vi "jVision.vi"() -> ()   [LabVIEW 2013]
uses:
  <vilib>/userDefined/High Color/IMAQdx.ctl
  Controls/States.ctl
  <vilib>/vision/driver/NI_Vision_Acquisition_Software.lvlib
  <resource>/objmgr/imaqdx.rc
panel:
  in  "Auto Clear":bool=TRUE
  out "User Notes File Name":path
  in  "Experiment Notes":string
  in  "Set Camera Properties":bool=TRUE
  in  "SyncOutSource":string(combo)="FreeRun"
  in  "SyncOutSelector":string(combo)="FrameStart"
  out "Max. Frame Rate":u32
  out "Cam Session":T1 caption="Session Out"
  in  "File Name Prefix":string="Rawdata "
  in  "File Path":path=path "E:/Rawdata"
  in  "Width":u32=1920 min=1 max=1920
  in  "Height":u32=1080 min=1 max=1080
  out "Stopped":bool
  in  "Exp. Time (S)":u32=60
  out "Frames to Acquire":u32
  in  "Set Frame Rate":u32=25 max=60
  in  "Start":bool
  out "Exp Time":dbl caption="Elapsed Time (s)"
  out "Frame Rate":dbl format="%#_4f"
  in  "Camera ID":T1="cam1"
  out "Frames Acquired":i32
  out "JVision - Release F":T2(plugin-control)
  in  "Stop Button":bool
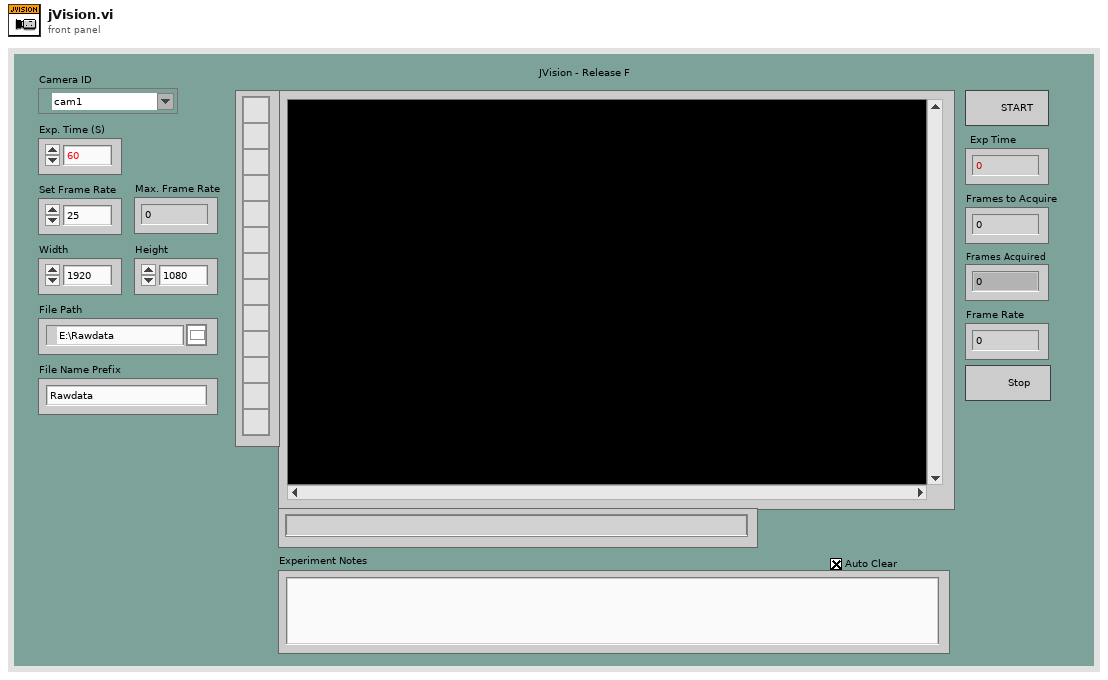
[diagram p1: front panel]
types:
  T1 = typedef "IMAQdx.ctl" = refnum<k21>
  T2 = typedef "IMAQ Image.ctl" = refnum<image>
  T3 = typedef "States.ctl" = enum16{"Initialize", "Wait for Start", "Set Param", "Initialize Acquisition", "Run Acquisition", "Stop"}
  T4 = enum16{"open", "replace", "create", "open or create", "replace or create", "replace or create with confirmation"}
  T5 = typedef "Image Type" = u32
  T6 = enum8{"Enabled", "Disabled", "Disabled and Grayed Out"}
  T7 = typedef "AviRefnum.ctl" = refnum<k1>
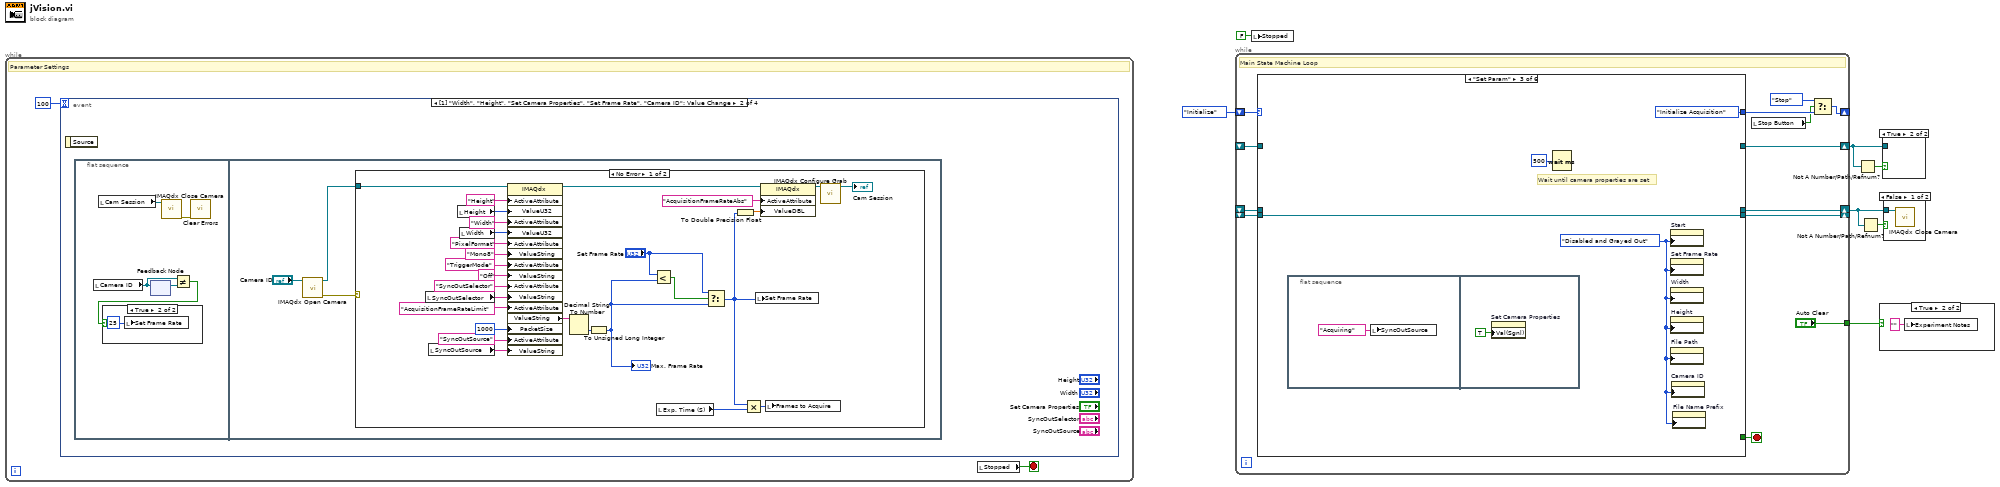
[diagram p0: block diagram]
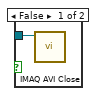
[diagram p4: hidden frame]
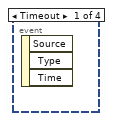
[diagram p5: hidden frame]
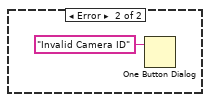
[diagram p7: hidden frame]
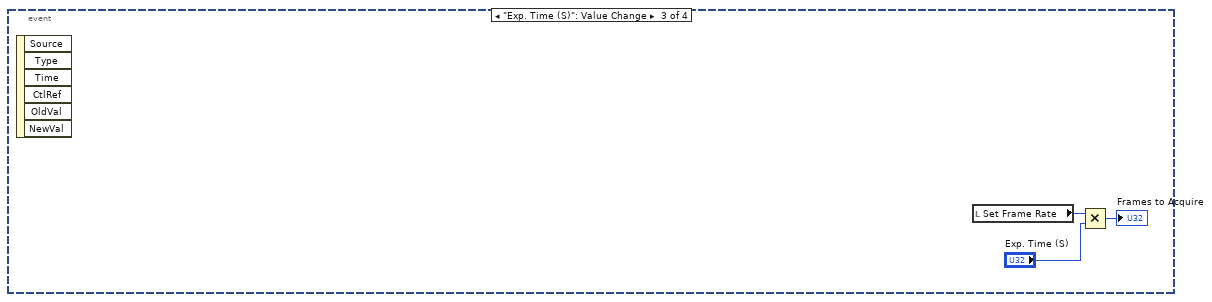
[diagram p8: hidden frame]
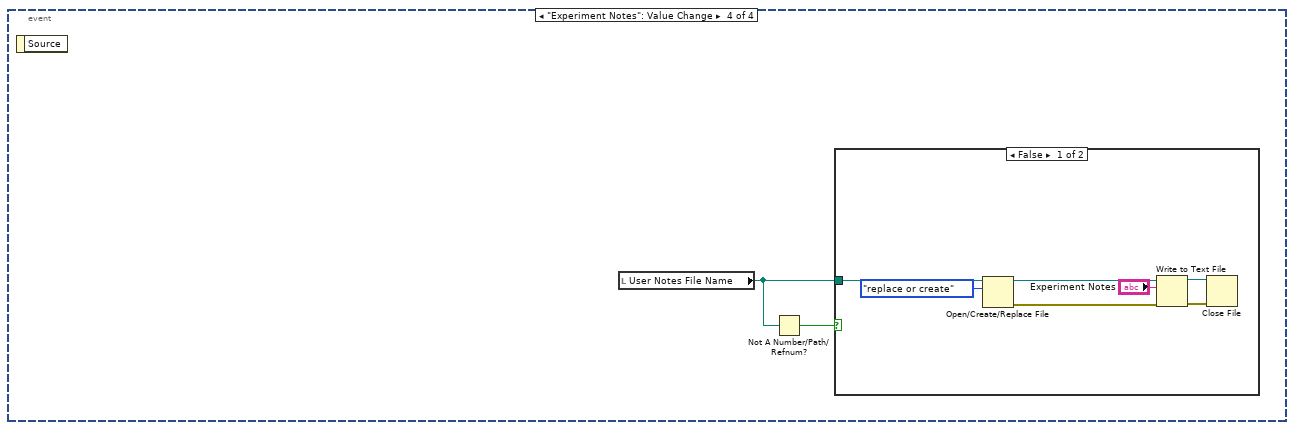
[diagram p9: hidden frame]
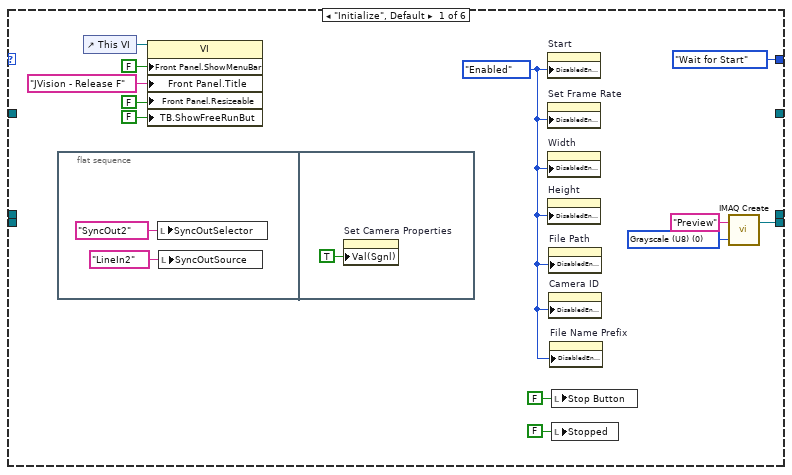
[diagram p11: hidden frame]
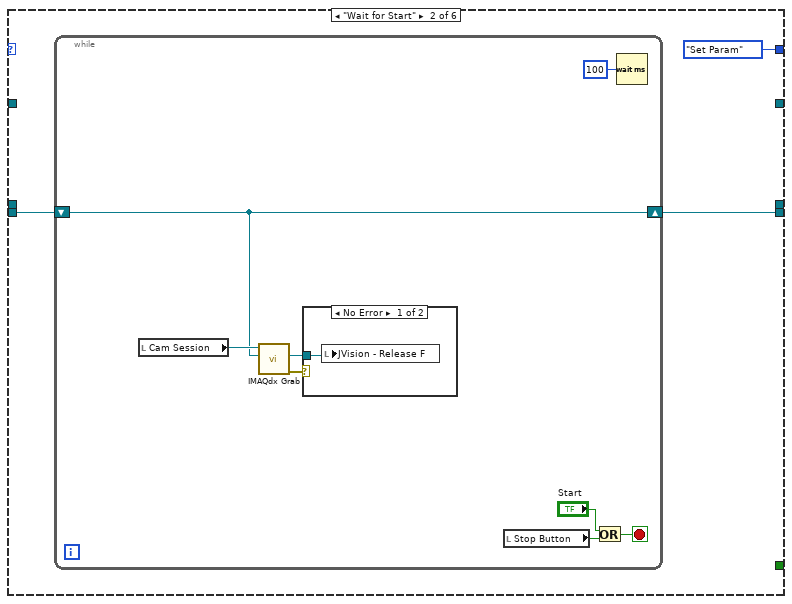
[diagram p12: hidden frame]
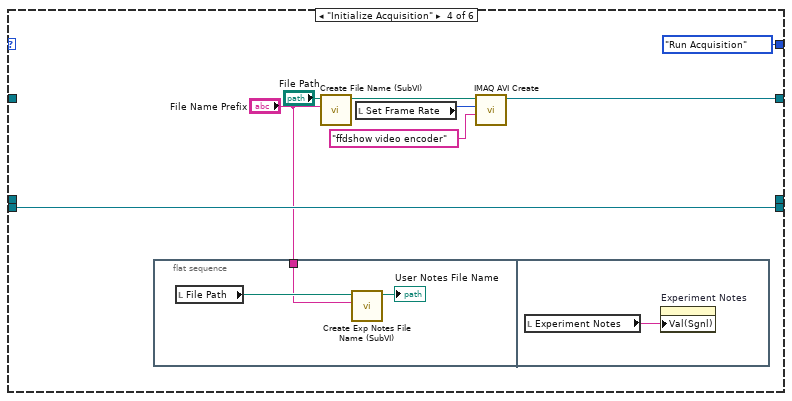
[diagram p14: hidden frame]
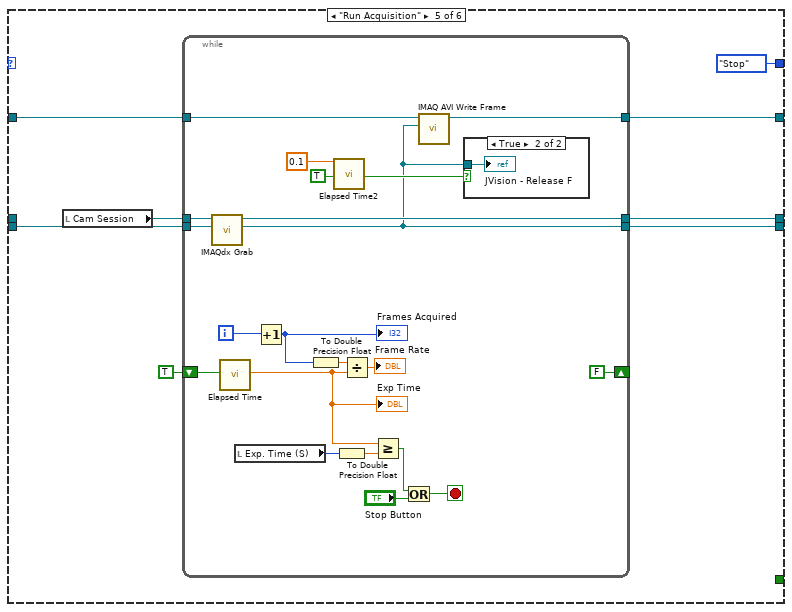
[diagram p15: hidden frame]
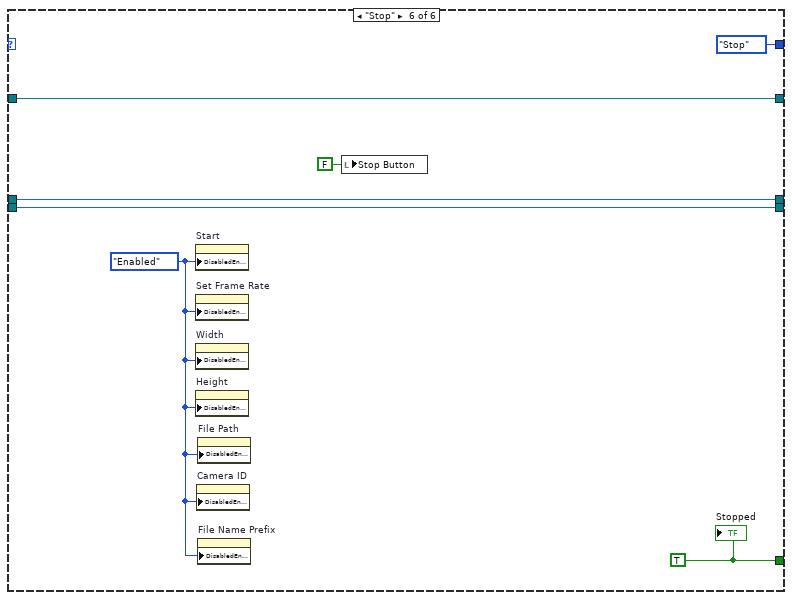
[diagram p17: hidden frame]
diagram:
  n1 = while {
    stop <- w9 stop-if-true
    # "Parameter Settings"
    n2 = event shown="[1] \"Width\", \"Height\", \"Set Camera Properties\", \"Set Frame Rate\", \"Camera ID\": Value Change" {
      selector: _ -> [_ _ _ _]
      dyn-events: _ -> [_ _ _ _]
      timeout: 100 -> [_ _ _ _]
      event Timeout {
        n3 = event-data() -> ()  [unwired: 1 in, 3 out]
      }
      event "Width", "Height", "Set Camera Properties", "Set Frame Rate": Value Change {
        n4 = event-data() -> ()  [unwired: 1 in, 1 out]
        n5 = flat-sequence {
          frame #0 {
            n6 = local read "Camera ID"() -> (w11:T1)
            n7 = local read "Cam Session"() -> (w13:T1)
            n8 = feedback #1() -> (w12:T1)  [unwired: 1 in]
            n9 = feedback-in #1(w11) -> ()
            n10 = call <vilib>:"IMAQdx Close Camera.vi"("Session In"=w13) -> ("error out"=w14:errorcluster)  [unwired: 10 in]
            n11 = Not Equal?(x=w11, y=w12) -> (x != y?=w10:bool)
            n12 = case shown="True" w10 {
              frame False {
              }
              frame True {
                n13 = local write "Set Frame Rate"(u32 25 ("Set Frame Rate")) -> ()
              }
            }
            n14 = call <vilib>:"Clear Errors.vi"("error in (no error)"=w14) -> ()  [unwired: 6 in, 1 out]
          }
          frame #1 {
            n15 = call <vilib>:"IMAQdx Open Camera.vi"("Session In"="Camera ID") -> ("error out"=w17:errorcluster, "Session Out"=w16:T1)  [unwired: 9 in]
            n16 = case shown="No Error" w17 {
              tunnel: w16 -> [w19 _]
              frame No Error {
                n17 = local read "SyncOutSelector"() -> (w25:string)
                n18 = local read "SyncOutSource"() -> (w24:string)
                n19 = local read "Height"() -> (w44:u32)
                n20 = local read "Width"() -> (w43:u32)
                n21 = property class="IMAQdx"(reference=w19, "ActiveAttribute"="Height", "ValueU32"=w44, "ActiveAttribute"="Width", "ValueU32"=w43, "ActiveAttribute"="PixelFormat", "ValueString"="Mono8" ("ActiveAttribute"), "ActiveAttribute"="TriggerMode", "ValueString"="Off", "ActiveAttribute"="SyncOutSelector", "ValueString"=w25, "ActiveAttribute"="AcquisitionFrameRateLimit", "PacketSize"=u32 1000, "ActiveAttribute"="SyncOutSource", "ValueString"=w24) -> (reference out=w32:T1, "ValueString"=w36:string)  [unwired: 1 in, 1 out]
                n22 = Decimal String To Number(string=w36) -> (number=w37:i32)  [unwired: 2 in, 1 out]
                n23 = To Unsigned Long Integer(number=w37) -> (unsigned 32bit integer=w28:u32)
                "Max. Frame Rate" <- w28
                n24 = Less?(x="Set Frame Rate", y=w28) -> (x < y?=w34:bool)
                n25 = local read "Exp. Time (S)"() -> (w22:u32)
                n26 = Select(t="Set Frame Rate", s=w34, f=w28) -> (s? t:f=w21:u32)
                n27 = To Double Precision Float(number=w21) -> (double precision float=w29:dbl)
                n28 = Multiply(x=w21, y=w22) -> (x*y=w23:u32)
                n29 = local write "Set Frame Rate"(w21) -> ()
                n30 = property class="IMAQdx"(reference=w32, "ActiveAttribute"="AcquisitionFrameRateAbs", "ValueDBL"=w29) -> (reference out=w31:T1)  [unwired: 1 in, 1 out]
                n31 = local write "Frames to Acquire"(w23) -> ()
                n32 = call <vilib>:"IMAQdx Configure Grab.vi"("Session In"=w31) -> ("Session Out"=→"Cam Session":T1)  [unwired: 9 in, 1 out]
              }
              frame Error {
                n33 = One Button Dialog(message="Invalid Camera ID") -> ()  [unwired: 1 in, 1 out]
              }
            }
          }
        }
      }
      event "Exp. Time (S)": Value Change {
        n34 = event-data() -> ()  [unwired: 1 in, 6 out]
        n35 = local read "Set Frame Rate"() -> (w50:u32)
        n36 = Multiply(x=w50, y="Exp. Time (S)") -> (x*y=→"Frames to Acquire":u32)
      }
      event "Experiment Notes": Value Change {
        n37 = event-data() -> ()  [unwired: 1 in, 1 out]
        n38 = local read "User Notes File Name"() -> (w52:path)
        n39 = Not A Number/Path/Refnum?(number/path/refnum=w52) -> (NaN/Path/Refnum?=w51:bool)
        n40 = case shown="False" w51 {
          tunnel: w52 -> [w53 _]
          frame False {
            n41 = Open/Create/Replace File(file path (use dialog)=w53, operation (0:open)=T4."replace or create") -> (refnum out=w57:refnum<file>, error out=w58:errorcluster)  [unwired: 4 in, 1 out]
            n42 = Write to Text File(file (use dialog)=w57, text="Experiment Notes", error in=w58) -> (refnum out=w54:refnum<file>, error out=w55:errorcluster)  [unwired: 1 in, 1 out]
            n43 = Close File(refnum=w54, error in=w55) -> ()  [unwired: 2 out]
          }
          frame True {
          }
        }
      }
    }
    n44 = local read "Stopped"() -> (w9:bool)
  }
  n45 = while {
    shift-right: [w63] -> _
    shift-left: States."Initialize" ("Enum") -> [w71]
    shift-right: [w70] -> _
    shift-left: _ -> [w69]
    shift-right: [w68] -> w4
    shift-left: _ -> [w67]
    shift-right: [w66] -> w6
    shift-left: _ -> [w65]
    tunnel: ["Auto Clear"] -> w1
    stop <- w64 stop-if-true
    # "Main State Machine Loop"
    n46 = case shown="\"Set Param\"" w71 {
      tunnel: [States."Wait for Start" ("Enum") States."Set Param" ("Enum") States."Initialize Acquisition" ("Enum") States."Run Acquisition" ("Enum") States."Stop" ("Enum") States."Stop" ("Enum")] -> w72
      tunnel: [w81 w88 w102 w107 w119 w152] -> w70
      tunnel: w69 -> [_ w89 w102 w107 w123 w152]
      tunnel: [_ _ _ _ w120 w151] -> w68
      tunnel: w67 -> [_ _ _ _ _ w151]
      tunnel: [_ _ _ w108 w121 w153] -> w66
      tunnel: w65 -> [_ _ _ _ w124 w153]
      tunnel: [_ _ _ _ _ w149] -> w64
      frame "Initialize", Default {
        w83 = T5 0 items=["Grayscale (U8)", "Grayscale (I16)", "Grayscale (SGL)", "Complex (CSG)", "RGB (U32)", "HSL (U32)", "RGB (U64)", "Grayscale (U16)"] ("Image Type")
        w80 = T6."Enabled" ("Disabled")
        n47 = flat-sequence {
          frame #0 {
            n48 = local write "SyncOutSelector"("SyncOut2" ("SyncOutSelector")) -> ()
            n49 = local write "SyncOutSource"("LineIn2" ("SyncOutSource")) -> ()
          }
          frame #1 {
            n50 = property on="Set Camera Properties" class="Bool (strict)"("Val(Sgnl)"=TRUE ("Value (Signaling)")) -> ()  [unwired: 2 in, 2 out]
          }
        }
        n51 = control-ref of="This VI"() -> (w79:refnum<vi>)
        n52 = property class="VI"(reference=w79, "Front Panel.ShowMenuBar"=FALSE ("Front Panel Window:Show Menu Bar"), "Front Panel.Title"="JVision - Release F" ("Front Panel Window:Title"), "Front Panel.Resizeable"=FALSE ("Front Panel Window:Resizable"), "TB.ShowFreeRunBut"=FALSE ("Tool Bar:Show Free Run Button")) -> ()  [unwired: 1 in, 2 out]
        n53 = property on="Start" class="Bool"("DisabledEnum"=w80) -> ()  [unwired: 2 in, 2 out]
        n54 = property on="Set Frame Rate" class="DigNum (strict)"("DisabledEnum"=w80) -> ()  [unwired: 2 in, 2 out]
        n55 = property on="Width" class="DigNum (strict)"("DisabledEnum"=w80) -> ()  [unwired: 2 in, 2 out]
        n56 = property on="Height" class="DigNum (strict)"("DisabledEnum"=w80) -> ()  [unwired: 2 in, 2 out]
        n57 = property on="File Path" class="Path"("DisabledEnum"=w80) -> ()  [unwired: 2 in, 2 out]
        n58 = property on="Camera ID" class="IMAQdx (strict)"("DisabledEnum"=w80) -> ()  [unwired: 2 in, 2 out]
        n59 = property on="File Name Prefix" class="Str"("DisabledEnum"=w80) -> ()  [unwired: 2 in, 2 out]
        n60 = local write "Stop Button"(FALSE ("Stop Button")) -> ()
        n61 = local write "Stopped"(FALSE ("Stopped")) -> ()
        n62 = call "IMAQ Create"("Image Name"="Preview", "Image Type"=w83) -> ("New Image"=w81:T2)  [unwired: 3 in, 1 out]
      }
      frame "Wait for Start" {
        n63 = while {
          shift-right: [w91] -> w88
          shift-left: w89 -> [w91]
          stop <- w95 stop-if-true
          n64 = local read "Cam Session"() -> (w94:T1)
          n65 = call <vilib>:"IMAQdx Grab.vi"("Image In"=w91, "Session In"=w94) -> ("error out"=w93:errorcluster, "Image Out"=w92:T2)  [unwired: 6 in, 2 out]
          n66 = case shown="No Error" w93 {
            tunnel: w92 -> [w99 _]
            frame No Error {
              n67 = local write "JVision - Release F"(w99) -> ()
            }
            frame Error {
            }
          }
          n68 = local read "Stop Button"() -> (w96:bool)
          n69 = Or(x="Start", y=w96) -> (x .or. y?=w95:bool)
          n70 = Wait (ms)(milliseconds to wait=u32 100) -> ()  [unwired: 1 out]
        }
      }
      frame "Set Param" {
        w101 = T6."Disabled and Grayed Out" ("Disabled")
        # "Wait until camera properties are set"
        n71 = flat-sequence {
          frame #0 {
            n72 = local write "SyncOutSource"("Acquiring" ("SyncOutSource")) -> ()
          }
          frame #1 {
            n73 = property on="Set Camera Properties" class="Bool (strict)"("Val(Sgnl)"=TRUE ("Value (Signaling)")) -> ()  [unwired: 2 in, 2 out]
          }
        }
        n74 = Wait (ms)(milliseconds to wait=u32 500) -> ()  [unwired: 1 out]
        n75 = property on="Start" class="Bool"("DisabledEnum"=w101) -> ()  [unwired: 2 in, 2 out]
        n76 = property on="Set Frame Rate" class="DigNum (strict)"("DisabledEnum"=w101) -> ()  [unwired: 2 in, 2 out]
        n77 = property on="Width" class="DigNum (strict)"("DisabledEnum"=w101) -> ()  [unwired: 2 in, 2 out]
        n78 = property on="Height" class="DigNum (strict)"("DisabledEnum"=w101) -> ()  [unwired: 2 in, 2 out]
        n79 = property on="File Path" class="Path"("DisabledEnum"=w101) -> ()  [unwired: 2 in, 2 out]
        n80 = property on="Camera ID" class="IMAQdx (strict)"("DisabledEnum"=w101) -> ()  [unwired: 2 in, 2 out]
        n81 = property on="File Name Prefix" class="Str"("DisabledEnum"=w101) -> ()  [unwired: 2 in, 2 out]
      }
      frame "Initialize Acquisition" {
        n82 = flat-sequence {
          tunnel: "File Name Prefix" -> [w114]
          frame #0 {
            n83 = local read "File Path"() -> (w116:path)
            n84 = call "Create Exp Notes File Name (SubVI).vi"("File Name Prefix"=w114, "File Path"=w116) -> ("File Name"=→"User Notes File Name":path)  [unwired: 9 in]
          }
          frame #1 {
            n85 = local read "Experiment Notes"() -> (w117:string)
            n86 = property on="Experiment Notes" class="Str"("Val(Sgnl)"=w117) -> ()  [unwired: 2 in, 2 out]
          }
        }
        n87 = call "Create File Name (SubVI).vi"("File Name Prefix"="File Name Prefix", "File Path"="File Path") -> ("File Name"=w111:path)  [unwired: 9 in]
        n88 = local read "Set Frame Rate"() -> (w113:u32)
        n89 = call "IMAQ AVI Create"("Compression Filter"="ffdshow video encoder", "Frames Per Second"=w113, "AVI Path"=w111) -> ("Avi Refnum"=w108:T7)  [unwired: 7 in, 1 out]
      }
      frame "Run Acquisition" {
        n90 = local read "Cam Session"() -> (w118:T1)
        n91 = while {
          tunnel: w118 -> [w145]
          tunnel: w123 -> [w144]
          tunnel: [w143] -> w120
          shift-right: [FALSE] -> _
          shift-left: TRUE -> [w140]
          tunnel: w124 -> [w129]
          tunnel: [w130] -> w121
          tunnel: [w128] -> w119
          i -> [w126]
          stop <- w142 stop-if-true
          n92 = call <vilib>:"IMAQdx Grab.vi"("Image In"=w144, "Session In"=w145) -> ("Image Out"=w128:T2, "Session Out"=w143:T1)  [unwired: 6 in, 2 out]
          n93 = call "Elapsed Time"("Reset"=w140) -> ("Elapsed Time (s)"=w131:dbl)  [unwired: 11 in, 7 out]
          "Exp Time" <- w131
          n94 = local read "Exp. Time (S)"() -> (w136:u32)
          n95 = Increment(x=w126) -> (x+1=w127:i32)
          "Frames Acquired" <- w127
          n96 = To Double Precision Float(number=w127) -> (double precision float=w137:dbl)
          n97 = call "Elapsed Time2"("Time Target (s)"=0.1, "Auto Reset"=TRUE) -> ("Time has Elapsed"=w133:bool)  [unwired: 10 in, 7 out]
          n98 = To Double Precision Float(number=w136) -> (double precision float=w135:dbl)
          n99 = Divide(x=w137, y=w131) -> (x/y=→"Frame Rate":dbl)
          n100 = Greater Or Equal?(x=w131, y=w135) -> (x >= y?=w141:bool)
          n101 = Or(x=w141, y="Stop Button") -> (x .or. y?=w142:bool)
          n102 = call "IMAQ AVI Write Frame"("Image"=w128, "Avi Refnum"=w129) -> ("Avi Refnum (duplicate)"=w130:T7)  [unwired: 8 in, 1 out]
          n103 = case shown="True" w133 {
            tunnel: w128 -> [_ w147]
            frame False {
            }
            frame True {
              "JVision - Release F" <- w147
            }
          }
        }
      }
      frame "Stop" {
        w148 = T6."Enabled" ("Disabled")
        w149 = TRUE
        n104 = property on="Start" class="Bool"("DisabledEnum"=w148) -> ()  [unwired: 2 in, 2 out]
        n105 = property on="Set Frame Rate" class="DigNum (strict)"("DisabledEnum"=w148) -> ()  [unwired: 2 in, 2 out]
        n106 = property on="Width" class="DigNum (strict)"("DisabledEnum"=w148) -> ()  [unwired: 2 in, 2 out]
        n107 = property on="Height" class="DigNum (strict)"("DisabledEnum"=w148) -> ()  [unwired: 2 in, 2 out]
        n108 = property on="Camera ID" class="IMAQdx (strict)"("DisabledEnum"=w148) -> ()  [unwired: 2 in, 2 out]
        n109 = property on="File Path" class="Path"("DisabledEnum"=w148) -> ()  [unwired: 2 in, 2 out]
        n110 = property on="File Name Prefix" class="Str"("DisabledEnum"=w148) -> ()  [unwired: 2 in, 2 out]
        n111 = local write "Stop Button"(FALSE ("Stop Button")) -> ()
        "Stopped" <- w149
      }
    }
    n112 = local read "Stop Button"() -> (w62:bool)
    n113 = Select(t=States."Stop" ("Enum"), s=w62, f=w72) -> (s? t:f=w63:T3)
  }
  n114 = local write "Stopped"(FALSE ("Stopped")) -> ()
  n115 = Not A Number/Path/Refnum?(number/path/refnum=w6) -> (NaN/Path/Refnum?=w5:bool)
  n116 = Not A Number/Path/Refnum?(number/path/refnum=w4) -> (NaN/Path/Refnum?=w3:bool)
  n117 = case shown="True" w1 {
    frame False {
    }
    frame True {
      n118 = local write "Experiment Notes"("" ("Experiment Notes")) -> ()
    }
  }
  n119 = case shown="True" w5 {
    tunnel: w6 -> [w156 _]
    frame False {
      n120 = call "IMAQ AVI Close"("Avi Refnum"=w156) -> ()  [unwired: 10 in, 1 out]
    }
    frame True {
    }
  }
  n121 = case shown="False" w3 {
    tunnel: w4 -> [w157 _]
    frame False {
      n122 = call <vilib>:"IMAQdx Close Camera.vi"("Session In"=w157) -> ()  [unwired: 10 in, 1 out]
    }
    frame True {
    }
  }
